vi "test selector.vi"() -> ()   [LabVIEW 2014]
uses:
  Collector State.ctl
panel:
  out "data":T1
  out "x+1":i32
  in  "deleteShot":bool
  in  "undoLastShot":bool
  in  "RESET All":bool
  in  "saveShots":bool
  in  "readyClock":bool caption="Clock"
  in  "addShot":bool caption="RANGE SETUP must be selected before shots can be added."
  in  "reportV50":bool caption="Report"
  in  "clearShots":bool
  in  "reportV50_History":bool
  in  "nextShot":bool
  in  "processShots":bool caption="Proc Shots"
  in  "VsVr Report":bool caption="Report"
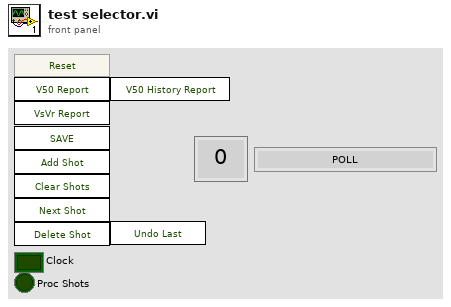
[diagram p1: front panel]
types:
  T1 = typedef "Collector State.ctl" = enum16{"POLL", "INITIALIZE", "V50 Report or GET Record", "VsVr Report", "SAVE SHOTS", "ADD SHOT", "CLEAR SHOTS", "NEXT SHOT", "DELETE SHOT", "READY CLOCK", "PROCESS SHOTS", "CHECK DAQ"}
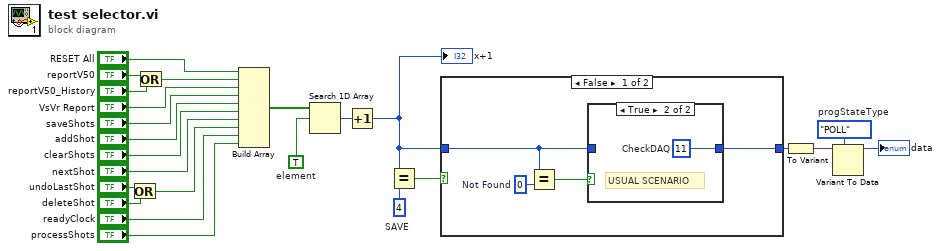
[diagram p0: block diagram]
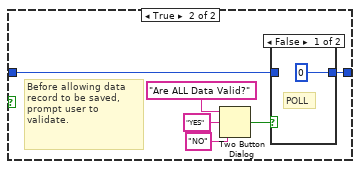
[diagram p3: hidden frame]
diagram:
  w9 = Collector_State."POLL"  # progStateType
  w8 = 4  # SAVE
  w17 = TRUE  # element
  n1 = Or(x="undoLastShot", y="deleteShot") -> (x .or. y?=w19:bool)
  n2 = Or(x="reportV50", y="reportV50_History") -> (x .or. y?=w13:bool)
  n3 = Build Array("RESET All", w13, "VsVr Report", "saveShots", "addShot", "clearShots", "nextShot", w19, "readyClock", "processShots") -> (w16:bool[])
  n4 = Search 1D Array(1D array=w16, element=w17) -> (index of element=w10:i32)  [unwired: 1 out]
  n5 = Increment(x=w10) -> (x+1=w5:i32)
  "x+1" <- w5
  n6 = Equal?(x=w5, y=w8) -> (x = y?=w6:bool)
  n7 = case shown="False" w6 {
    tunnel: w5 -> [w26 w32]
    tunnel: [w25 w31] -> w4
    frame False {
      w27 = 0  # Not Found
      n8 = Equal?(x=w26, y=w27) -> (x = y?=w28:bool)
      n9 = case shown="True" w28 {
        tunnel: w26 -> [w29 _]
        tunnel: [w29 w30] -> w25
        frame False {
        }
        frame True {
          w30 = 11  # CheckDAQ
          # "USUAL SCENARIO"
        }
      }
    }
    frame True {
      # "Before allowing data record to be saved,\nprompt user to validate."
      n10 = Two Button Dialog(message="Are ALL Data Valid?", 1:"NO" ("F button name (\"Cancel\")"), 2:"YES" ("T button name (\"OK\")")) -> (T button?=w33:bool)
      n11 = case shown="False" w33 {
        tunnel: [0 ("index of element") w38] -> w31
        tunnel: w32 -> [_ w38]
        frame False {
          # "POLL"
        }
        frame True {
        }
      }
    }
  }
  n12 = To Variant(anything=w4) -> (Variant=w7:variant)
  n13 = Variant To Data(type=w9, Variant=w7) -> (data=→"data":T1)  [unwired: 1 in, 1 out]
